vi "MSScript_Format_UpdAO.vi"(9 "ValueArray":string[](array[string]), 10 "TagArray":string[](array[string]), 11 "MSScript.lvclass":refnum<class "MSScript.lvclass">) -> (0 "ValueErrorArray":bool[](array[boolean]), 1 "TagErrorArray":bool[](array[boolean]), 2 "ParamErrorArray":bool[](array[boolean]), 3 "Data":variant, 4 "#ofParamError":bool)   [LabVIEW 2018, in "MSScript.lvclass"]
uses:
  MSScript.lvclass
  Ctl/MSEditorParam updAO.ctl
  MSScript_Transform_UIntArray.vi
  MSScript_Transform_EXTArray.vi
panel:
  in  "ParamValueType":T1={"func"=[0, 0, 0, 0], "val"=[0.0, 0.0, 0.0, 0.0]}
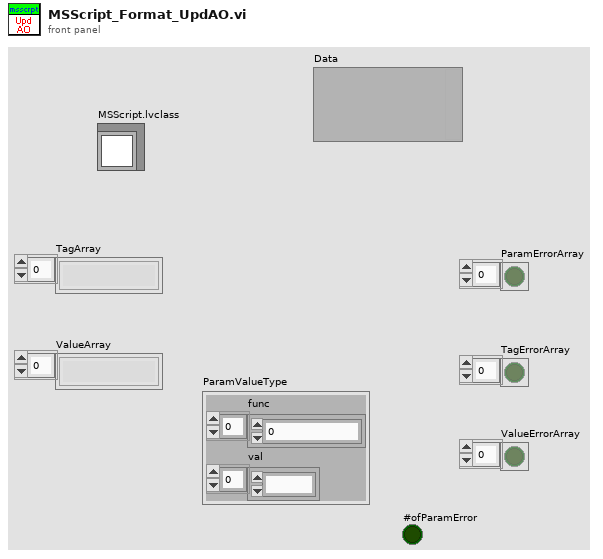
[diagram p1: front panel]
types:
  T1 = typedef "MSEditorParam updAO.ctl" = cluster{"func":u32[], "val":ext[]}
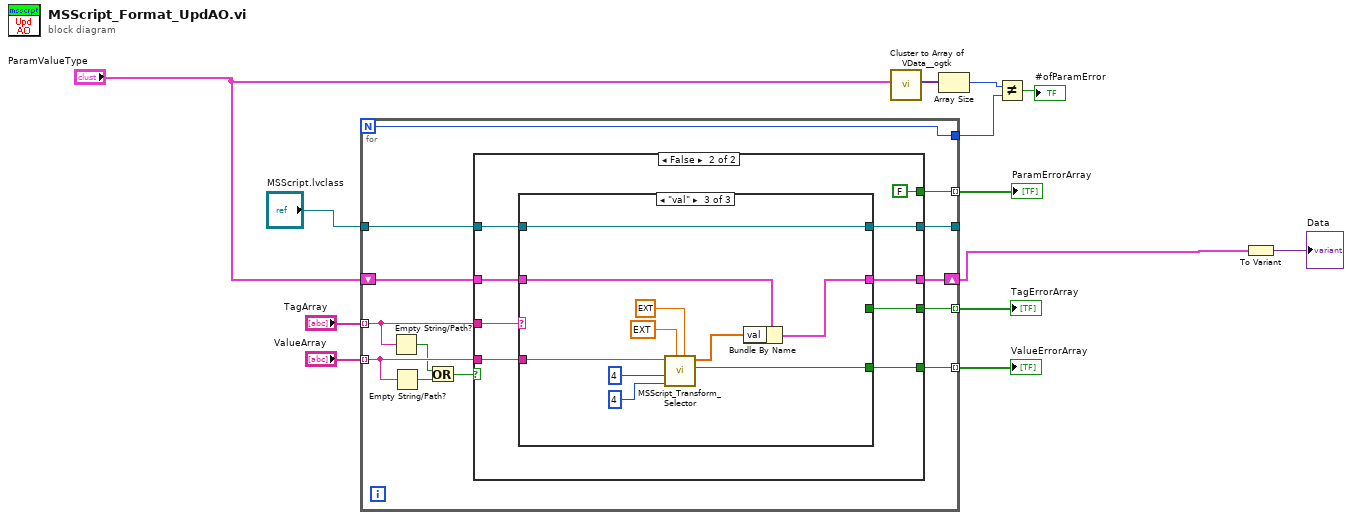
[diagram p0: block diagram]
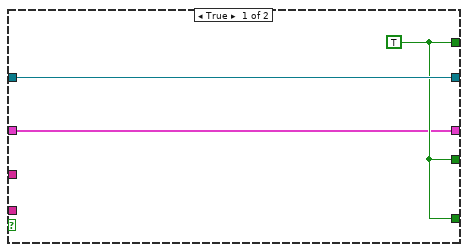
[diagram p2: hidden frame]
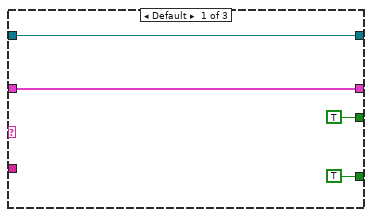
[diagram p3: hidden frame]
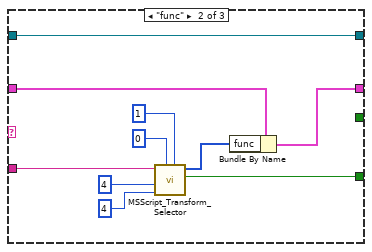
[diagram p4: hidden frame]
diagram:
  n1 = for {
    N -> [w14]
    tunnel: "TagArray" -> [w22] mode=indexing
    tunnel: "ValueArray" -> [w21] mode=indexing
    tunnel: [w26] -> w11 mode=indexing
    tunnel: "MSScript.lvclass" -> [w25]
    tunnel: [w24] -> w10 mode=indexing
    tunnel: [w23] -> _
    tunnel: [w17] -> w9 mode=indexing
    shift-right: [w15] -> w2
    shift-left: "ParamValueType" -> [w16]
    tunnel: [w14] -> w4
    n2 = Empty String/Path?(string/path=w22) -> (empty?=w19:bool)
    n3 = Empty String/Path?(string/path=w21) -> (empty?=w20:bool)
    n4 = Or(x=w19, y=w20) -> (x .or. y?=w18:bool)
    n5 = case shown="False" w18 {
      tunnel: [w28 w32] -> w26
      tunnel: w25 -> [w29 w37]
      tunnel: [w28 w33] -> w24
      tunnel: [w29 w30] -> w23
      tunnel: w22 -> [_ w35]
      tunnel: w21 -> [_ w34]
      tunnel: [w28 FALSE] -> w17
      tunnel: w16 -> [w27 w36]
      tunnel: [w27 w31] -> w15
      frame True {
        w28 = TRUE
      }
      frame False {
        n6 = case shown="\"val\"" w35 {
          tunnel: [TRUE _ _] -> w32
          tunnel: w37 -> [w40 w50 w60]
          tunnel: w34 -> [_ w51 w61]
          tunnel: [TRUE ("Value Error?") w52 w62] -> w33
          tunnel: [w40 w50 w60] -> w30
          tunnel: w36 -> [w39 w48 w58]
          tunnel: [w39 w47 w57] -> w31
          frame Default {
          }
          frame "func" {
            n7 = call-poly "MSScript_Transform_Selector.vi"("upper limit (18446744073709551615)"=u64 1 ("upper limit"), "lower limit (0)"=u64 0 ("lower limit"), "MinSize"=4, "MaxSize"=4, "Check_Str"=w51) -> ("Value Error?"=w52:bool, "Value Output"=w49:u64[])  [unwired: 4 in, 1 out]
            n8 = Bundle By Name(cluster=w48, "func"=w49) -> (w47:T1)
          }
          frame "val" {
            n9 = call-poly "MSScript_Transform_Selector.vi"("upper limit (Inf)"=ext 10.0 ("upper limit"), "lower limit (-Inf)"=ext -10.0 ("lower limit"), "MinSize"=4, "MaxSize"=4, "check_str"=w61) -> ("Value Error?"=w62:bool, "Value Output"=w59:ext[])  [unwired: 4 in, 1 out]
            n10 = Bundle By Name(cluster=w58, "val"=w59) -> (w57:T1)
          }
        }
      }
    }
  }
  "TagErrorArray" <- w11
  "ValueErrorArray" <- w10
  "ParamErrorArray" <- w9
  n11 = call <userlib>:"Cluster to Array of VData__ogtk.vi"("Cluster"="ParamValueType") -> ("Array of VData"=w7:variant[])  [unwired: 9 in, 1 out]
  n12 = Array Size(array=w7) -> (size(s)=w6:i32)
  n13 = Not Equal?(x=w6, y=w4) -> (x != y?=→"#ofParamError":bool)
  n14 = To Variant(anything=w2) -> (Variant=→"Data":variant)
